vi "OAT Output Buffered Data (Even Angle, N Chan).vi"(0 "even-angle signals":cluster{"r0":dbl, "dr":dbl, "Y":dbl[]}[](array[cluster]) {"r0" format="%.2p"; "dr" format="%.2p"; "Y" format="%.2f"}, 2 "reset? (F)":bool, 7 "even-angle position info":T1, 11 "error in (no error)":errorcluster, 12 "buffer settings":T2) -> (4 "buffered even-angle signals":cluster{"r0":dbl, "dr":dbl, "Y":dbl[]}[](array[cluster]) {"r0" format="%.2p"; "dr" format="%.2p"; "Y" format="%.2f"}, 8 "buffered even-angle position info":T1, 15 "error out":errorcluster)   [LabVIEW 2017, in "SoundVib_OAUtility.lvlib"]
doc: "Buffers the input signals and returns them in first-in first-out (FIFO) mode. Use <B>buffer settings</B> to set the buffer size and units. Each instance of this VI maintains its own state; use the N Waveforms instance of this VI to process an array of channels. Wire data to the <B>XY signal</B> input to determine the polymorphic instance to use or manually select the instance."
uses:
  <vilib>/addons/Sound and Vibration/Order Analysis/Utility/SoundVib_OAUtility.lvlib
  <vilib>/addons/Sound and Vibration/Order Analysis/Misc/OAT Position Info.ctl
  <vilib>/addons/Sound and Vibration/Order Analysis/Utility/SubVIs/oa_Buffer Settings.ctl
  <vilib>/addons/_NISVFA/_Shared subVIs/Common/svc_Get Array Subset (Index).vi
  <vilib>/addons/_NISVFA/_Shared subVIs/Common/svc_Coerce Index and Length.vi
  <vilib>/addons/_NISVFA/_Shared subVIs/Common/svc_Conditional Merge Error.vi
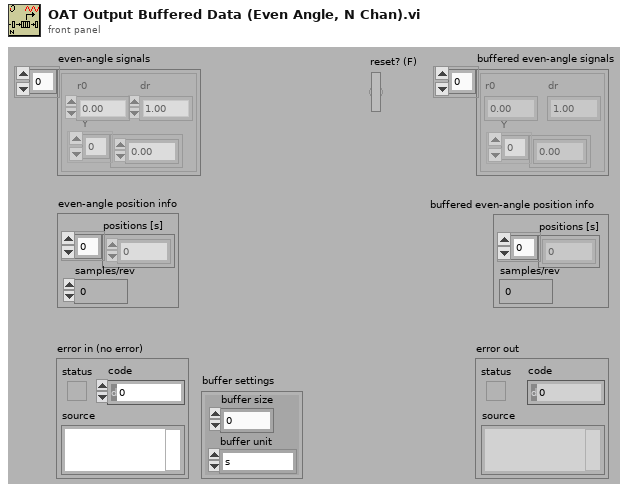
[diagram p1: front panel]
types:
  T1 = typedef "OAT Position Info.ctl" = cluster{"positions [s]":dbl[], "samples/rev":dbl}
  T2 = typedef "SoundVib_OAUtility.lvlib/oa_Buffer Settings.ctl" = cluster{"buffer size":dbl, "buffer unit":enum16{"s", "revolution", "# of samples"}}
  T3 = cluster{"positions [s]":dbl[], "samples/rev":dbl}
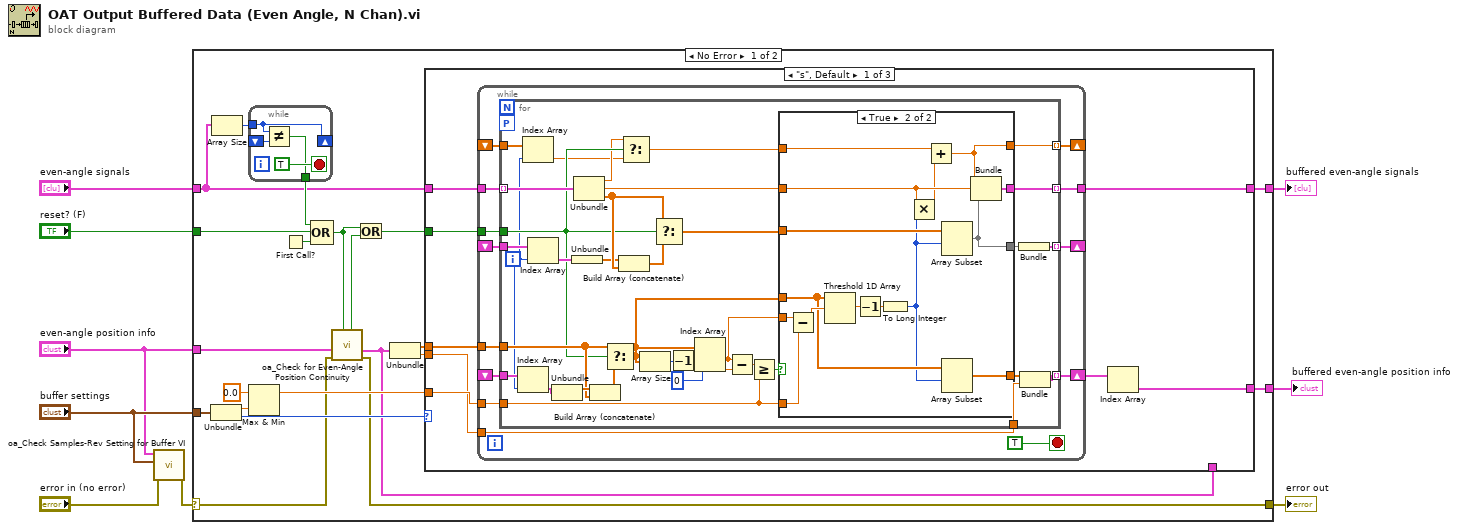
[diagram p0: block diagram]
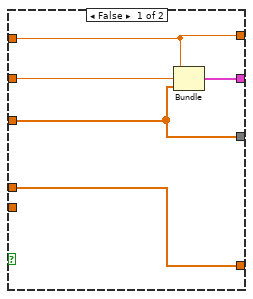
[diagram p2: hidden frame]
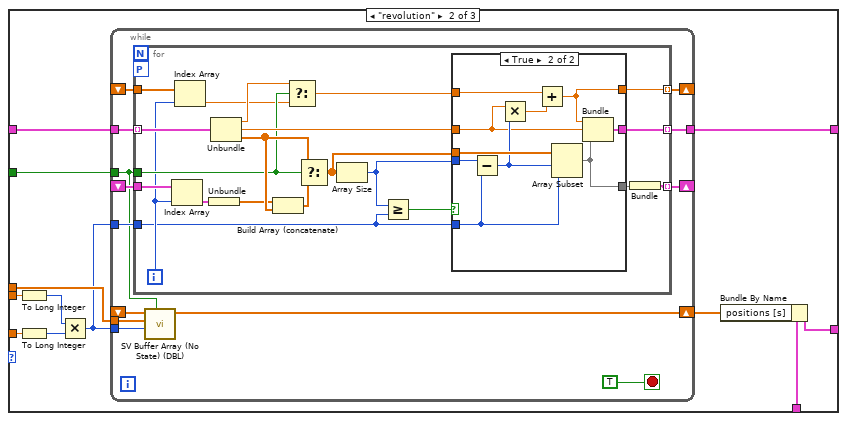
[diagram p3: hidden frame]
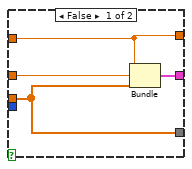
[diagram p4: hidden frame]
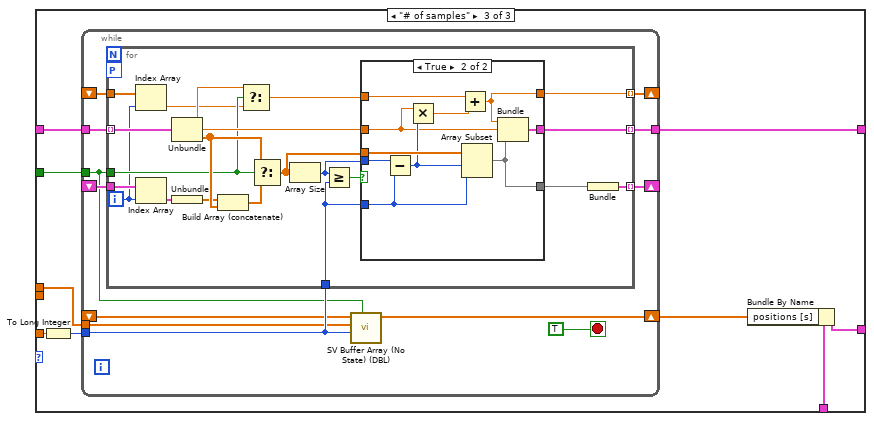
[diagram p5: hidden frame]
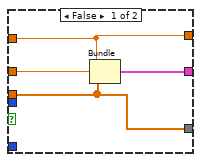
[diagram p6: hidden frame]
diagram:
  n1 = call <vilib>:"oa_Check Samples-Rev Setting for Buffer VI.vi"("error in (no error)"="error in (no error)", "buffer settings"="buffer settings", "position info"="even-angle position info") -> ("error out"=w5:errorcluster)  [unwired: 8 in]
  n2 = case shown="No Error" w5 {
    selector: w5 -> [w16 w227]
    tunnel: [w15 w227] -> w7
    tunnel: "buffer settings" -> [w30 _]
    tunnel: "even-angle signals" -> [w20 _]
    tunnel: "reset? (F)" -> [w22 _]
    tunnel: [w27 _] -> w6
    tunnel: "even-angle position info" -> [w19 _]
    tunnel: [w10 _] -> w1
    frame No Error {
      n3 = Unbundle(w30) -> ("buffer size"=w25:dbl, "buffer unit"=w26:enum16{"s", "revolution", "# of samples"})
      n4 = Array Size(array=w20) -> (size(s)=w24:i32)
      n5 = while {
        tunnel: w24 -> [w33]
        shift-right: [w33] -> _
        shift-left: _ -> [w34]
        tunnel: [w31] -> w23
        stop <- TRUE stop-if-true
        n6 = Not Equal?(x=w33, y=w34) -> (x != y?=w31:bool)
      }
      n7 = Max & Min(x=0.0, y=w25) -> (max(x,y)=w28:dbl)  [unwired: 1 out]
      n8 = First Call?() -> (First Call?: T/F=w21:bool)
      n9 = Compound Arithmetic op=OR(w23, w22, w21) -> (w17:bool)
      n10 = call <vilib>:"oa_Check for Even-Angle Position Continuity.vi"("reset in"=w17, "error in (no error)"=w16, "even-angle position info"=w19) -> ("error out"=w15:errorcluster, "even-angle position info dup"=w11:T1, "position not continuous"=w13:bool)  [unwired: 6 in]
      n11 = Or(x=w17, y=w13) -> (x .or. y?=w14:bool)
      n12 = Unbundle(w11) -> ("positions [s]"=w18:dbl[], "samples/rev"=w12:dbl)
      n13 = case shown="\"s\", Default" w26 {
        tunnel: w28 -> [w41 w120 w176]
        tunnel: w20 -> [w39 w122 w179]
        tunnel: w14 -> [w38 w121 w178]
        tunnel: [w40 w119 w177] -> w27
        tunnel: w18 -> [w42 w118 w174]
        tunnel: w12 -> [w37 w115 _]
        tunnel: w11 -> [_ w117 w172]
        tunnel: [w35 w111 w171] -> w10
        frame "s", Default {
          n14 = while {
            tunnel: w42 -> [w52]
            tunnel: w41 -> [w51]
            tunnel: [w55] -> w40
            tunnel: w39 -> [w49]
            shift-right: [w54] -> _
            shift-left: _ -> [w50]
            tunnel: w38 -> [w48]
            shift-right: [w47] -> w36
            shift-left: _ -> [w46]
            shift-right: [w45] -> _
            shift-left: _ -> [w44]
            tunnel: w37 -> [w43]
            stop <- TRUE stop-if-true
            n15 = for {
              tunnel: [w84] -> w55 mode=indexing
              tunnel: [w75] -> w54 mode=indexing
              tunnel: w52 -> [w65]
              tunnel: w51 -> [w81]
              tunnel: w50 -> [w77]
              tunnel: w49 -> [w79] mode=indexing
              tunnel: w48 -> [w63]
              tunnel: [w70] -> w47 mode=indexing
              tunnel: w46 -> [w69]
              tunnel: [w60] -> w45 mode=indexing
              tunnel: w44 -> [w59]
              tunnel: w43 -> [w56]
              workers-P: _ -> [_]
              i -> [w58]
              n16 = Index Array(array=w69, index=w58) -> (element=w67:T3)
              n17 = Index Array(array=w59, index=w58) -> (element=w57:dbl)
              n18 = Index Array(array=w77, index=w58) -> (element=w74:cluster{"Y":dbl[]})
              n19 = Unbundle(w67) -> ("positions [s]"=w66:dbl[])  [unwired: 1 out]
              n20 = Unbundle(w74) -> ("Y"=w73:dbl[])
              n21 = Unbundle(w79) -> ("r0"=w62:dbl, "dr"=w72:dbl, "Y"=w76:dbl[])
              n22 = Build Array (concatenate)(w66, w65) -> (w64:dbl[])
              n23 = Select(t=w65, s=w63, f=w64) -> (s? t:f=w68:dbl[])
              n24 = Build Array (concatenate)(w73, w76) -> (w80:dbl[])
              n25 = Select(t=w62, s=w63, f=w57) -> (s? t:f=w61:dbl)
              n26 = Array Size(array=w68) -> (size(s)=w90:i32)
              n27 = Select(t=w76, s=w63, f=w80) -> (s? t:f=w78:dbl[])
              n28 = Decrement(x=w90) -> (x-1=w89:i32)
              n29 = Index Array(array=w68, index #1=w89, index #2=0 ("index")) -> (element #1=w82:dbl, element #2=w87:dbl)
              n30 = Subtract(x=w82, y=w87) -> (x-y=w86:dbl)
              n31 = Greater Or Equal?(x=w86, y=w81) -> (x >= y?=w85:bool)
              n32 = case shown="True" w85 {
                tunnel: [w95 w106] -> w84
                tunnel: [w94 w104] -> w83
                tunnel: w68 -> [w92 w102]
                tunnel: w82 -> [_ w110]
                tunnel: w81 -> [_ w109]
                tunnel: w78 -> [w94 w105]
                tunnel: w72 -> [w93 w99]
                tunnel: w61 -> [w91 w98]
                tunnel: [w92 w101] -> w71
                tunnel: [w91 w96] -> w60
                frame False {
                  n33 = Bundle("r0"=w91, "dr"=w93, "Y"=w94) -> (w95:cluster{"r0":dbl, "dr":dbl, "Y":dbl[]})  [unwired: 1 in]
                }
                frame True {
                  n34 = Subtract(x=w110, y=w109) -> (x-y=w108:dbl)
                  n35 = Threshold 1D Array(2:w108, 3:w102) -> (0:w107:dbl)  [unwired: 1 in]
                  n36 = Decrement(x=w107) -> (x-1=w103:dbl)
                  n37 = To Long Integer(number=w103) -> (32bit integer=w100:i32)
                  n38 = Multiply(x=w99, y=w100) -> (x*y=w97:dbl)
                  n39 = Add(x=w98, y=w97) -> (x+y=w96:dbl)
                  n40 = Array Subset(array=w105, index=w100) -> (w104:dbl[])  [unwired: 1 in]
                  n41 = Array Subset(array=w102, index=w100) -> (w101:dbl[])  [unwired: 1 in]
                  n42 = Bundle(w96, "dr"=w99, w104) -> (w106:cluster{dbl, "dr":dbl, dbl[]})  [unwired: 1 in]
                }
              }
              n43 = Bundle("Y"=w83) -> (w75:cluster{"Y":dbl[]})  [unwired: 1 in]
              n44 = Bundle("positions [s]"=w71, "samples/rev"=w56) -> (w70:T3)  [unwired: 1 in]
            }
          }
          n45 = Index Array(array=w36) -> (element=w35:T3)  [unwired: 1 in]
        }
        frame "revolution" {
          n46 = To Long Integer(number=w115) -> (32bit integer=w114:i32)
          n47 = To Long Integer(number=w120) -> (32bit integer=w113:i32)
          n48 = Multiply(x=w114, y=w113) -> (x*y=w112:i32)
          n49 = while {
            tunnel: w122 -> [w135]
            shift-right: [w133] -> _
            shift-left: _ -> [w131]
            tunnel: w121 -> [w125]
            tunnel: w112 -> [w130]
            tunnel: [w132] -> w119
            shift-right: [w128] -> _
            shift-left: _ -> [w129]
            shift-right: [w127] -> w116
            shift-left: _ -> [w126]
            tunnel: w118 -> [w124]
            tunnel: w112 -> [w123]
            stop <- TRUE stop-if-true
            n50 = for {
              tunnel: w135 -> [w156] mode=indexing
              tunnel: w125 -> [w141]
              tunnel: [w148] -> w133 mode=indexing
              tunnel: [w153] -> w132 mode=indexing
              tunnel: w131 -> [w150]
              tunnel: w130 -> [w136]
              tunnel: w129 -> [w143]
              tunnel: [w139] -> w128 mode=indexing
              workers-P: _ -> [_]
              i -> [w137]
              n51 = Index Array(array=w150, index=w137) -> (element=w147:cluster{"Y":dbl[]})
              n52 = Index Array(array=w143, index=w137) -> (element=w138:dbl)
              n53 = Unbundle(w147) -> ("Y"=w146:dbl[])
              n54 = Unbundle(w156) -> ("r0"=w142:dbl, "dr"=w145:dbl, "Y"=w149:dbl[])
              n55 = Build Array (concatenate)(w146, w149) -> (w151:dbl[])
              n56 = Select(t=w142, s=w141, f=w138) -> (s? t:f=w140:dbl)
              n57 = Select(t=w149, s=w141, f=w151) -> (s? t:f=w155:dbl[])
              n58 = Array Size(array=w155) -> (size(s)=w144:i32)
              n59 = Greater Or Equal?(x=w144, y=w136) -> (x >= y?=w152:bool)
              n60 = case shown="True" w152 {
                tunnel: w155 -> [w158 w170]
                tunnel: w144 -> [_ w168]
                tunnel: [w158 w166] -> w154
                tunnel: [w160 w169] -> w153
                tunnel: w136 -> [_ w167]
                tunnel: w145 -> [w159 w163]
                tunnel: w140 -> [w157 w165]
                tunnel: [w157 w161] -> w139
                frame False {
                  n61 = Bundle("r0"=w157, "dr"=w159, "Y"=w158) -> (w160:cluster{"r0":dbl, "dr":dbl, "Y":dbl[]})  [unwired: 1 in]
                }
                frame True {
                  n62 = Subtract(x=w168, y=w167) -> (x-y=w164:i32)
                  n63 = Multiply(x=w163, y=w164) -> (x*y=w162:dbl)
                  n64 = Add(x=w165, y=w162) -> (x+y=w161:dbl)
                  n65 = Array Subset(array=w170, index=w164, length=w167) -> (w166:dbl[])
                  n66 = Bundle(w161, "dr"=w163, w166) -> (w169:cluster{dbl, "dr":dbl, dbl[]})  [unwired: 1 in]
                }
              }
              n67 = Bundle("Y"=w154) -> (w148:cluster{"Y":dbl[]})  [unwired: 1 in]
            }
            n68 = call <vilib>:"SV Buffer Array (No State) (DBL).vi"("clear buffer (False)"=w125, "buffer length  [samples] (-1 = unlimited)"=w123, "Y"=w124, "buffer in"=w126) -> ("buffer out"=w127:dbl[])  [unwired: 7 in]
          }
          n69 = Bundle By Name(cluster=w117, "positions [s]"=w116) -> (w111:T1)
        }
        frame "# of samples" {
          n70 = To Long Integer(number=w176) -> (32bit integer=w175:i32)
          n71 = while {
            tunnel: w179 -> [w191]
            shift-right: [w189] -> _
            shift-left: _ -> [w187]
            tunnel: w178 -> [w181]
            tunnel: w175 -> [w184]
            tunnel: [w188] -> w177
            shift-right: [w185] -> _
            shift-left: _ -> [w186]
            shift-right: [w183] -> w173
            shift-left: _ -> [w182]
            tunnel: w174 -> [w180]
            stop <- TRUE stop-if-true
            n72 = for {
              tunnel: w191 -> [w212] mode=indexing
              tunnel: w184 -> [w192]
              tunnel: w181 -> [w198]
              tunnel: [w202] -> w189 mode=indexing
              tunnel: [w208] -> w188 mode=indexing
              tunnel: w187 -> [w205]
              tunnel: w186 -> [w197]
              tunnel: [w195] -> w185 mode=indexing
              workers-P: _ -> [_]
              i -> [w193]
              n73 = Index Array(array=w197, index=w193) -> (element=w194:dbl)
              n74 = Index Array(array=w205, index=w193) -> (element=w204:cluster{"Y":dbl[]})
              n75 = Unbundle(w212) -> ("r0"=w199:dbl, "dr"=w200:dbl, "Y"=w203:dbl[])
              n76 = Unbundle(w204) -> ("Y"=w201:dbl[])
              n77 = Build Array (concatenate)(w201, w203) -> (w206:dbl[])
              n78 = Select(t=w199, s=w198, f=w194) -> (s? t:f=w196:dbl)
              n79 = Select(t=w203, s=w198, f=w206) -> (s? t:f=w211:dbl[])
              n80 = Array Size(array=w211) -> (size(s)=w210:i32)
              n81 = Greater Or Equal?(x=w210, y=w192) -> (x >= y?=w207:bool)
              n82 = case shown="True" w207 {
                tunnel: w211 -> [w216 w226]
                tunnel: w192 -> [_ w224]
                tunnel: w210 -> [_ w225]
                tunnel: [w216 w223] -> w209
                tunnel: [w215 w222] -> w208
                tunnel: w200 -> [w214 w219]
                tunnel: w196 -> [w213 w221]
                tunnel: [w213 w217] -> w195
                frame False {
                  n83 = Bundle("r0"=w213, "dr"=w214, "Y"=w216) -> (w215:cluster{"r0":dbl, "dr":dbl, "Y":dbl[]})  [unwired: 1 in]
                }
                frame True {
                  n84 = Subtract(x=w225, y=w224) -> (x-y=w220:i32)
                  n85 = Multiply(x=w219, y=w220) -> (x*y=w218:dbl)
                  n86 = Add(x=w221, y=w218) -> (x+y=w217:dbl)
                  n87 = Array Subset(array=w226, index=w220, length=w224) -> (w223:dbl[])
                  n88 = Bundle(w217, "dr"=w219, w223) -> (w222:cluster{dbl, "dr":dbl, dbl[]})  [unwired: 1 in]
                }
              }
              n89 = Bundle("Y"=w209) -> (w202:cluster{"Y":dbl[]})  [unwired: 1 in]
            }
            n90 = call <vilib>:"SV Buffer Array (No State) (DBL).vi"("clear buffer (False)"=w181, "buffer length  [samples] (-1 = unlimited)"=w184, "Y"=w180, "buffer in"=w182) -> ("buffer out"=w183:dbl[])  [unwired: 7 in]
          }
          n91 = Bundle By Name(cluster=w172, "positions [s]"=w173) -> (w171:T1)
        }
      }
    }
    frame Error {
    }
  }
  "error out" <- w7
  "buffered even-angle signals" <- w6
  "buffered even-angle position info" <- w1
